vi "directory.vi"() -> ()   [LabVIEW 2022 SP3]
panel:
  out "Application Directory":path
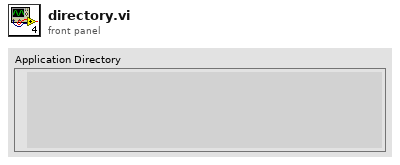
[diagram p1: front panel]
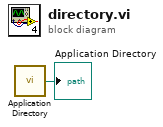
[diagram p0: block diagram]
diagram:
  n1 = call <vilib>:"Application Directory.vi"() -> ("Application Directory"=→"Application Directory":path)
